vi "Update Graph Legend.vi"(11 "UI Data in":refnum<class "Settings UI.lvclass">) -> (3 "UI Data out":refnum<class "Settings UI.lvclass">)   [LabVIEW 2020, in "Output Sequencer.lvlib" / "Settings UI.lvclass"]
uses:
  Settings UI.lvclass
  Settings UI.lvclass/Settings UI.ctl
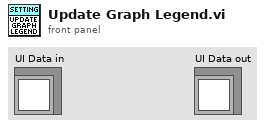
[diagram p1: front panel]
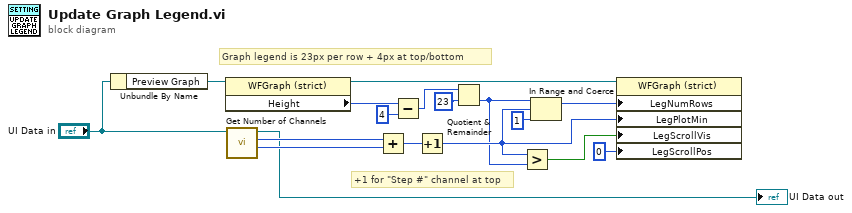
[diagram p0: block diagram]
diagram:
  # "+1 for \"Step #\" channel at top"
  # "Graph legend is 23px per row + 4px at top/bottom"
  n1 = Unbundle By Name("UI Data in") -> ("Preview Graph"=w1:refnum<vi>)
  n2 = property class="WFGraph (strict)"(reference=w1) -> (reference out=w6:refnum<vi>, "Height"=w12:u32)  [unwired: 1 in, 1 out]
  n3 = call "Get Number of Channels.vi"("UI Data In"="UI Data in") -> ("Num of Digital Channels"=w4:i32, "Num of Analog Channels"=w5:i32, "UI Data out"=→"UI Data out":refnum<class "Settings UI.lvclass">)  [unwired: 7 in, 1 out]
  n4 = Add(x=w5, y=w4) -> (x+y=w16:i32)
  n5 = Subtract(x=w12, y=u32 4) -> (x-y=w10:u32)
  n6 = Increment(x=w16) -> (x+1=w17:i32)
  n7 = Quotient & Remainder(x=w10, y=u32 23) -> (floor(x/y)=w8:u32)  [unwired: 1 out]
  n8 = Greater?(x=w17, y=w8) -> (0:w13:bool)
  n9 = In Range and Coerce(upper limit=w8, x=w17, lower limit=1) -> (coerced(x)=w14:u32)  [unwired: 1 out]
  n10 = property class="WFGraph (strict)"(reference=w6, "LegNumRows"=w14, "LegPlotMin"=w17, "LegScrollVis"=w13, "LegScrollPos"=u32 0 ("Legend:Scroll Position")) -> ()  [unwired: 1 in, 2 out]
